vi "locate seq channel by name.vi"(8 "error in":errorcluster, 10 "channel name":string, 11 "engine configuration in":refnum<class "base TBM sequencer configuration.lvclass">) -> (0 "error out":errorcluster, 2 "channel descriptor":refnum<class "TBM channel.lvclass">, 3 "engine configuration out":refnum<class "base TBM sequencer configuration.lvclass">)   [LabVIEW 2014, in "base TBM sequencer configuration.lvclass"]
uses:
  base TBM sequencer configuration.lvclass
  <vilib>/NI/Tag Bus Module Framework/channel/TBM channel.lvclass
  base TBM sequencer configuration.lvclass/base TBM sequencer configuration.ctl
  <vilib>/NI/Tag Bus/tag/tag descriptor.lvclass/tag descriptor.ctl
  <vilib>/NI/Tag Bus/tag/read tag name.vi
  <vilib>/NI/Tag Bus/tag/tag descriptor.lvclass
  <vilib>/NI/Configuration Framework/NISE_CEF_TreeControl.lvlib
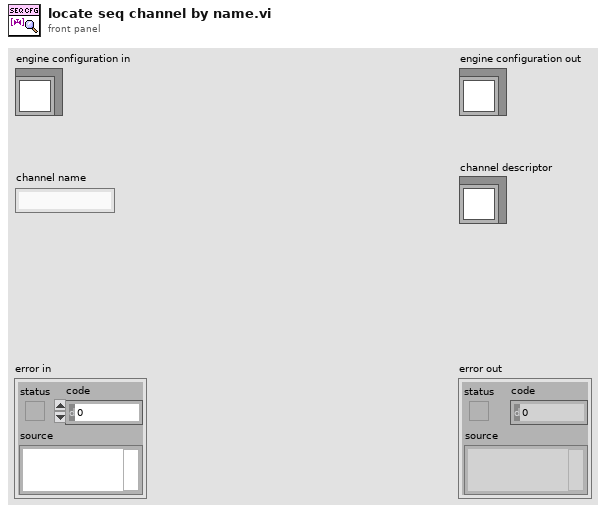
[diagram p1: front panel]
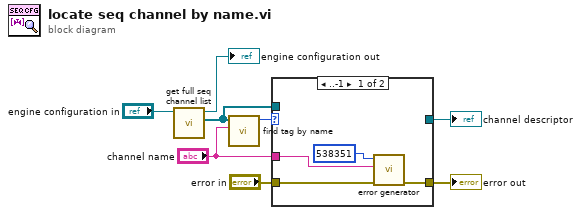
[diagram p0: block diagram]
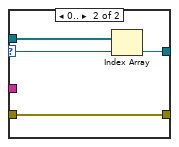
[diagram p2: hidden frame]
diagram:
  n1 = call "get full seq channel list.vi"("engine configuration in"="engine configuration in") -> ("seq channel list"=w6:refnum<class "TBM channel.lvclass">[], "engine configuration out"=→"engine configuration out":refnum<class "base TBM sequencer configuration.lvclass">)  [unwired: 9 in]
  n2 = call <vilib>:"find tag by name.vi"("name"="channel name", "tags in"=w6) -> ("index"=w4:i32)  [unwired: 9 in]
  n3 = case shown="..-1" w4 {
    selector: w4 -> [_ w14]
    tunnel: w6 -> [_ w16]
    tunnel: [_ w15] -> w5
    tunnel: "error in" -> [w11 w13]
    tunnel: [w12 w13] -> w2
    tunnel: "channel name" -> [w9 _]
    frame ..-1 {
      n4 = call <vilib>:"error generator.vi"("error in"=w11, "append error message"=w9, "error code (0)"=538351) -> ("error out"=w12:errorcluster)  [unwired: 6 in]
    }
    frame 0.. {
      n5 = Index Array(array=w16, index=w14) -> (element=w15:refnum<class "TBM channel.lvclass">)
    }
  }
  "error out" <- w2
  "channel descriptor" <- w5
